vi "Get Shooter LUT.vi"() -> (2 "Info":cluster{"Min Velocity":i32, "Max Velocity":i32}, 3 "LUT Out":i32[](array[numeric]))   [LabVIEW 2025]
panel:
  in  "Outputs":cluster{i32, i32}
  in  "Shooter LUT":i32[](array[numeric])=[0, 9500, 10500, 12500, 14000]
  out "Max Velocity":i32
  out "Min Velocity":i32
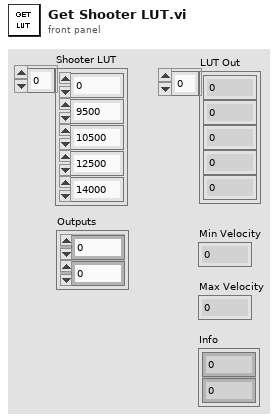
[diagram p1: front panel]
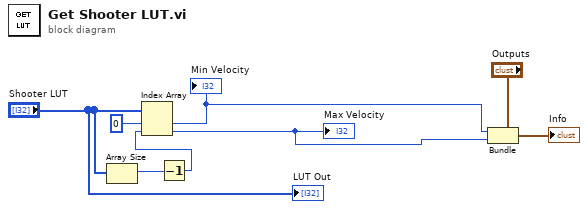
[diagram p0: block diagram]
diagram:
  n1 = Array Size(array="Shooter LUT") -> (size(s)=w7:i32)
  n2 = Decrement(x=w7) -> (x-1=w4:i32)
  n3 = Index Array(array="Shooter LUT", index #1=0 ("index"), index #2=w4) -> (element #1=w6:i32, element #2=w3:i32)
  "Min Velocity" <- w6
  "Max Velocity" <- w3
  n4 = Bundle(cluster="Outputs", w6, w3) -> (→"Info":cluster{i32, i32})
  "LUT Out" <- "Shooter LUT"
